vi "Mod_OFDM_bits_Generation_per_Frame.vi"(0 "Parameters per Ofdm Symbol":T1 {"Data Source"."Data Source"."Register Initial State" format="%08x"}, 7 "Initial SEED IN":u32[](array[numeric]), 11 "error in (no error)":errorcluster) -> (4 "Bits Generated":i8[](array[numeric]), 8 "Parameters per Ofdm Symbol":T1 {"Data Source"."Data Source"."Register Initial State" format="%08x"}, 15 "error out":errorcluster)   [LabVIEW 2010]
doc: "For each OFDM Symbol in the Frame bits are generated depending on the data sources assigned to the sub carriers and the configuration settings of the data sources."
uses:
  Controls(Type_DEf)/Parameters per Ofdm Symbol.ctl
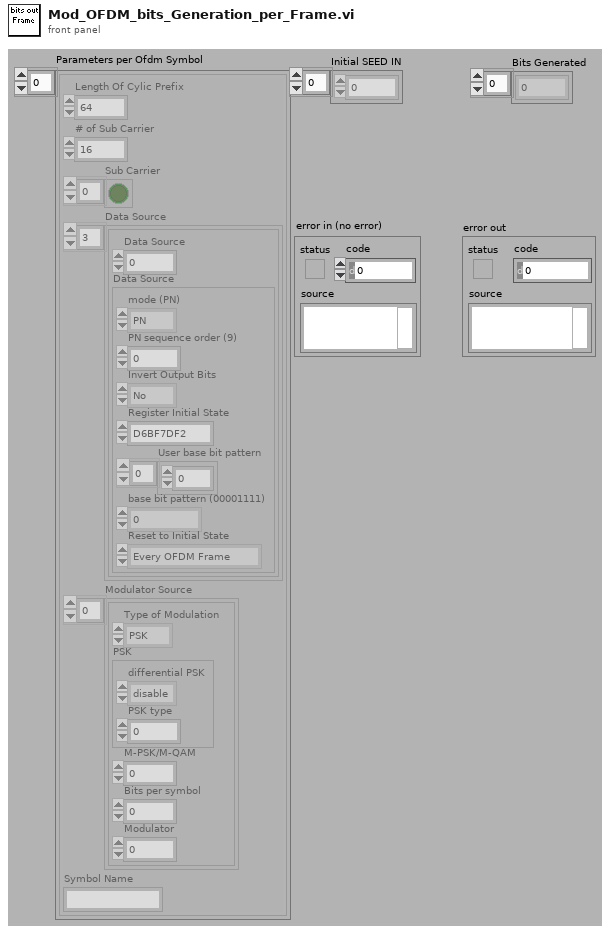
[diagram p1: front panel]
types:
  T1 = typedef "Parameters per Ofdm Symbol.ctl" = cluster{"Length Of Cylic Prefix":i32, "# of Sub Carrier":i32, "Sub Carrier":bool[], "Data Source":cluster{"Data Source":u16, "Data Source":cluster{"mode (PN)":enum16{"PN", "pattern", "user"}, "PN sequence order (9)":i32, "Invert Output Bits":enum16{"No", "Yes"}, "Register Initial State":u32, "User base bit pattern":i8[], "base bit pattern (00001111)":enum16{"0", "1", "01", "0011", "00001111"}, "Reset to Initial State":enum16{"Every OFDM Frame", "Every OFDM Symbol", "Every Sub Carrier"}}}[], "Modulator Source":cluster{"Type of Modulation":enum16{"PSK", "QAM"}, "PSK":cluster{"differential PSK":enum16{"disable", "enable"}, "PSK type":u16}, "M-PSK/M-QAM":i32, "Bits per symbol":i32, "Modulator":u16}[], "Symbol Name":string}[]
  T2 = cluster{"Type of Modulation":enum16{"PSK", "QAM"}, "PSK":cluster{"differential PSK":enum16{"disable", "enable"}, "PSK type":u16}, "M-PSK/M-QAM":i32, "Bits per symbol":i32, "Modulator":u16}[]
  T3 = cluster{"Data Source":u16, "Data Source":cluster{"mode (PN)":enum16{"PN", "pattern", "user"}, "PN sequence order (9)":i32, "Invert Output Bits":enum16{"No", "Yes"}, "Register Initial State":u32, "User base bit pattern":i8[], "base bit pattern (00001111)":enum16{"0", "1", "01", "0011", "00001111"}, "Reset to Initial State":enum16{"Every OFDM Frame", "Every OFDM Symbol", "Every Sub Carrier"}}}[]
  T4 = enum16{"Every OFDM Frame", "Every OFDM Symbol", "Every Sub Carrier"}
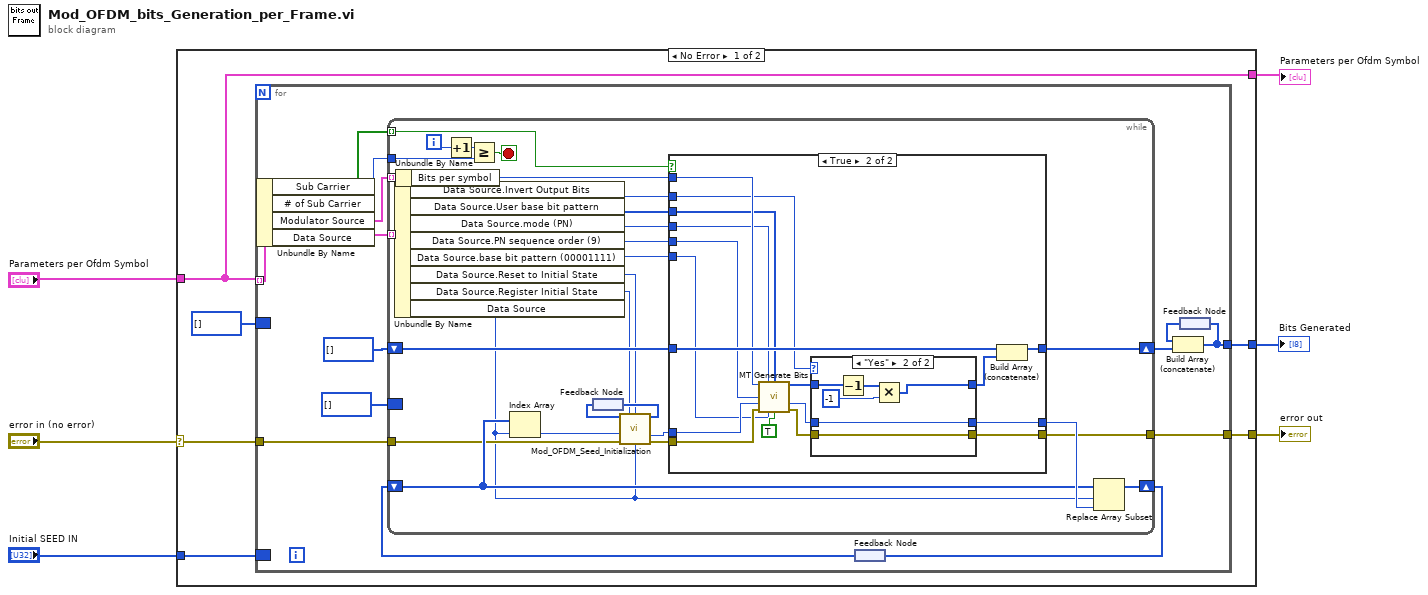
[diagram p0: block diagram]
diagram:
  n1 = case shown="No Error" "error in (no error)" {
    selector: "error in (no error)" -> [w11 w84]
    tunnel: [w12 w84] -> w6
    tunnel: "Parameters per Ofdm Symbol" -> [w10 _]
    tunnel: [w10 _] -> w3
    tunnel: "Initial SEED IN" -> [w9 _]
    tunnel: [w7 _] -> w1
    frame No Error {
      n2 = for {
        tunnel: w11 -> [w26]
        tunnel: [w25] -> w12
        tunnel: w10 -> [w23] mode=indexing
        tunnel: [w13] -> w7
        border: w9 -> [_]
        border: i8[] [] -> [_]
        n3 = Unbundle By Name(w23) -> ("Sub Carrier"=w16:bool[], "# of Sub Carrier"=w18:i32, "Modulator Source"=w17:T2, "Data Source"=w22:T3)
        n4 = feedback #1() -> (w19:u32[])
        n5 = while {
          tunnel: w18 -> [w45]
          shift-right: [w50] -> w20
          shift-left: w19 -> [w49]
          shift-right: [w46] -> w15
          shift-left: i8[] [] -> [w48]
          tunnel: w26 -> [w38]
          tunnel: [w47] -> w25
          tunnel: w16 -> [w44] mode=indexing
          tunnel: w22 -> [w43] mode=indexing
          tunnel: w17 -> [w42] mode=indexing
          border: i8[] [] -> [_]
          i -> [w54]
          stop <- w52 stop-if-true
          n6 = Unbundle By Name(w43) -> ("Data Source.Invert Output Bits"=w27:enum16{"No", "Yes"}, "Data Source.User base bit pattern"=w32:i8[], "Data Source.mode (PN)"=w31:enum16{"PN", "pattern", "user"}, "Data Source.PN sequence order (9)"=w30:i32, "Data Source.base bit pattern (00001111)"=w29:enum16{"0", "1", "01", "0011", "00001111"}, "Data Source.Reset to Initial State"=w33:T4, "Data Source.Register Initial State"=w34:u32, "Data Source"=w28:u16)
          n7 = Unbundle By Name(w42) -> ("Bits per symbol"=w41:i32)
          n8 = Increment(x=w54) -> (x+1=w53:i32)
          n9 = Greater Or Equal?(x=w53, y=w45) -> (x >= y?=w52:bool)
          n10 = Index Array(array=w49, index=w28) -> (element=w40:u32)
          n11 = feedback #2() -> (w35:i8[])
          n12 = call "Mod_OFDM_Seed_Initialization.vi"("Data Sources"=w35, "Register Initial State"=w34, "Data Source.Reset to Initial State"=w33, "Seed IN"=w40, "error in (no error)"=w38, "Data Source"=w28) -> ("Data Sources"=w36:i8[], "Seed OUT"=w39:i32, "error out"=w37:errorcluster)  [unwired: 7 in]
          n13 = feedback-in #2(w36) -> ()
          n14 = case shown="True" w44 {
            tunnel: [w57 w59] -> w51
            tunnel: w39 -> [w57 w74]
            tunnel: [w56 w72] -> w46
            tunnel: w48 -> [w56 w73]
            tunnel: w37 -> [w55 w71]
            tunnel: [w55 w60] -> w47
            tunnel: w41 -> [_ w69]
            tunnel: w29 -> [_ w68]
            tunnel: w30 -> [_ w67]
            tunnel: w31 -> [_ w66]
            tunnel: w32 -> [_ w65]
            tunnel: w27 -> [_ w64]
            frame False {
            }
            frame True {
              n15 = call <vilib>:"MT Generate Bits.vi"("total bits (128)"=w69, "mode (PN)"=w66, "user base bit pattern"=w65, "PN sequence order (9)"=w67, "seed in (0xD6BF7DF2)"=w74, "error in (no error)"=w71, "base bit pattern (00001111)"=w68, "reset? (T)"=TRUE) -> ("output bit stream"=w63:i8[], "seed out (PN Mode)"=w61:i32, "error out"=w62:errorcluster)  [unwired: 5 in]
              n16 = case shown="\"Yes\"" w64 {
                tunnel: w63 -> [w77 w81]
                tunnel: w62 -> [w75 w83]
                tunnel: w61 -> [w76 w82]
                tunnel: [w77 w78] -> w58
                tunnel: [w76 w82] -> w59
                tunnel: [w75 w83] -> w60
                frame "No", Default {
                }
                frame "Yes" {
                  n17 = Decrement(x=w81) -> (x-1=w80:i8[])
                  n18 = Multiply(x=w80, y=-1) -> (x*y=w78:i32[])
                }
              }
              n19 = Build Array (concatenate)(w73, w58) -> (w72:i32[])
            }
          }
          n20 = Replace Array Subset(array=w49, new element=w51, index=w28) -> (w50:u32[])
        }
        n21 = feedback-in #1(w20) -> ()
        n22 = feedback #3() -> (w14:i32[])
        n23 = Build Array (concatenate)(w14, w15) -> (w13:i32[])
        n24 = feedback-in #3(w13) -> ()
      }
    }
    frame Error {
    }
  }
  "error out" <- w6
  "Bits Generated" <- w1
  "Parameters per Ofdm Symbol" <- w3
